vi "MakeHTMLLink.vi"(1 "Link Target":string, 2 "Link Text":string) -> (0 "HTML Link":string)   [LabVIEW 2019, in "ArgosLib.lvlib"]
uses:
  ArgosLib.lvlib
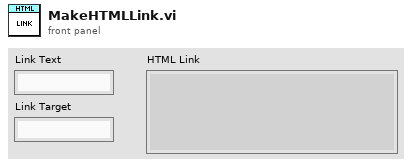
[diagram p1: front panel]
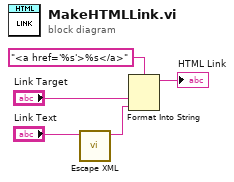
[diagram p0: block diagram]
diagram:
  n1 = call <vilib>:"Escape XML.vi"("XML String In"="Link Text") -> ("XML String Out"=w1:string)  [unwired: 9 in, 1 out]
  n2 = Format Into String(format string="<a href='%s'>%s</a>", "Link Target", w1) -> (resulting string=→"HTML Link":string)  [unwired: 2 in, 1 out]
